vi "Read Geodes.vi"(8 "error in (no error)":errorcluster, 11 "Blueprint in":refnum<class "Blueprint.lvclass">) -> (0 "error out":errorcluster, 2 "Geodes":u64, 3 "Blueprint out":refnum<class "Blueprint.lvclass">)   [LabVIEW 2021, in "d19.lvlib" / "Blueprint.lvclass"]
uses:
  Blueprint.lvclass
  Blueprint.lvclass/Blueprint.ctl
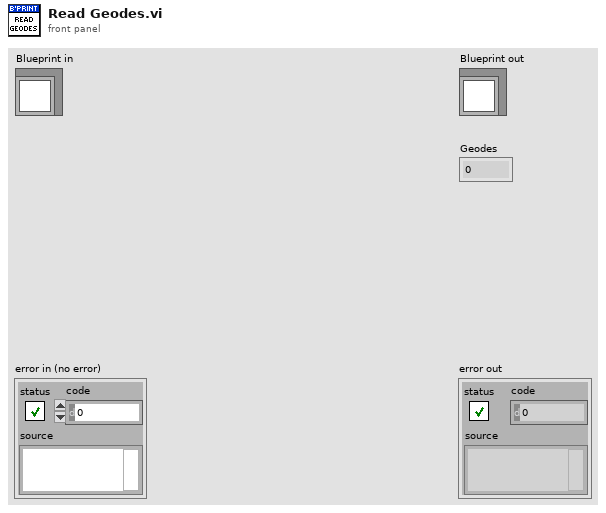
[diagram p1: front panel]
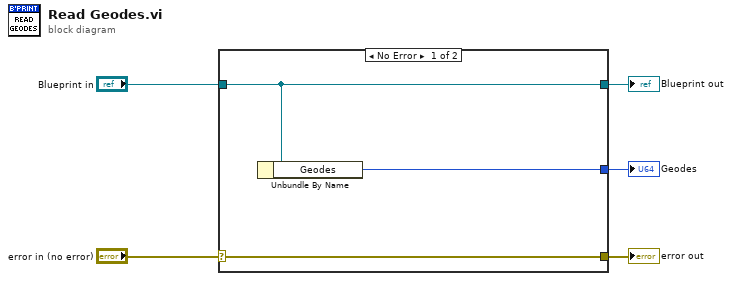
[diagram p0: block diagram]
diagram:
  n1 = case shown="No Error" "error in (no error)" {
    selector: "error in (no error)" -> [w8 w9]
    tunnel: [w8 w9] -> w4
    tunnel: [w7 w10] -> w2
    tunnel: "Blueprint in" -> [w7 w10]
    tunnel: [w6 _] -> w1
    frame No Error {
      n2 = Unbundle By Name(w7) -> ("Geodes"=w6:i64)
    }
    frame Error {
    }
  }
  "error out" <- w4
  "Blueprint out" <- w2
  "Geodes" <- w1
